vi "Do Done Template.vi"(1 "Init":bool, 5 "Do":bool) -> (6 "Done":bool)   [LabVIEW 2019]
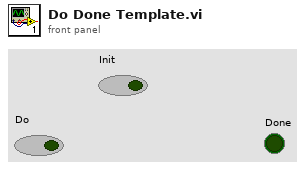
[diagram p1: front panel]
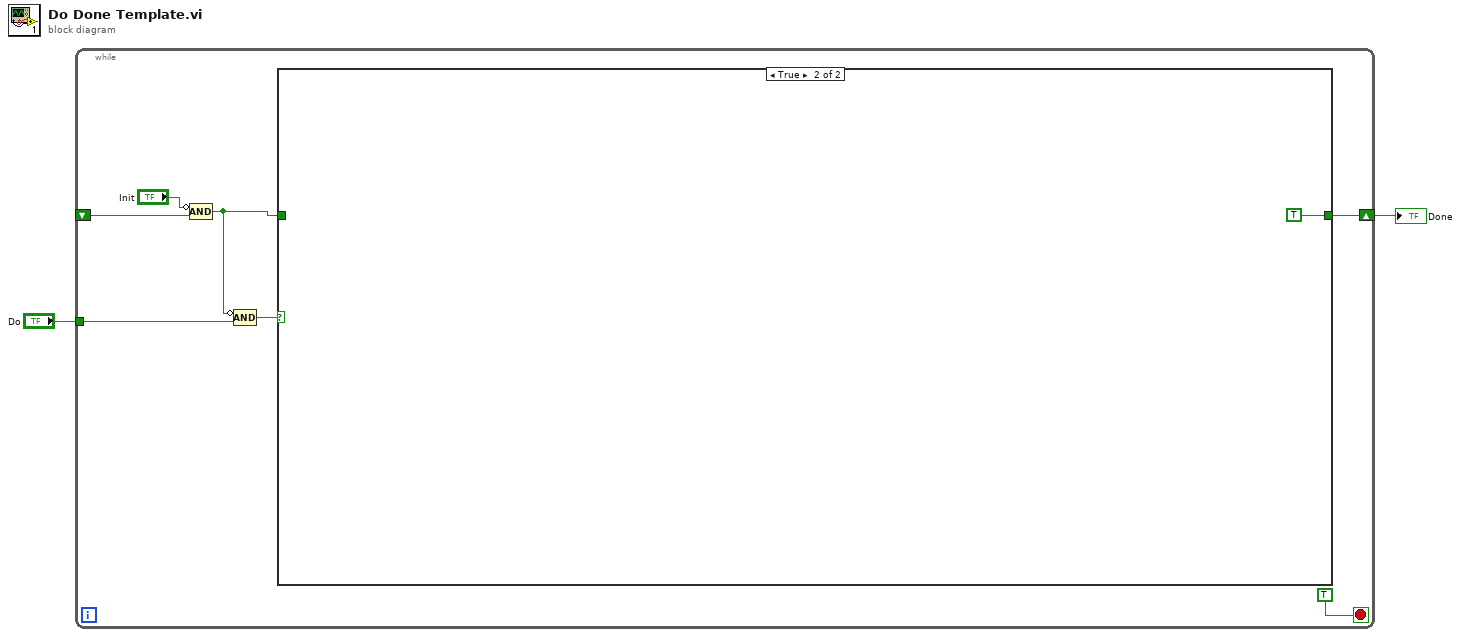
[diagram p0: block diagram]
diagram:
  n1 = while {
    tunnel: "Do" -> [w8]
    shift-right: [w6] -> w1
    shift-left: _ -> [w5]
    stop <- TRUE stop-if-true
    n2 = Compound Arithmetic op=AND(invert "Init", w5) -> (w4:bool)
    n3 = Compound Arithmetic op=AND(invert w4, w8) -> (w7:bool)
    n4 = case shown="True" w7 {
      tunnel: [w10 TRUE] -> w6
      tunnel: w4 -> [w10 _]
      frame False {
      }
      frame True {
      }
    }
  }
  "Done" <- w1
